vi "Write Move Enum_.vi"(8 "error in (no error)":errorcluster, 10 "Move Enum?":bool, 11 "Multi Column Listbox in":refnum<class "Multi Column Listbox.lvclass">) -> (0 "error out":errorcluster, 3 "Multi Column Listbox out":refnum<class "Multi Column Listbox.lvclass">)   [LabVIEW 2013]
uses:
  Multi Column Listbox.lvclass
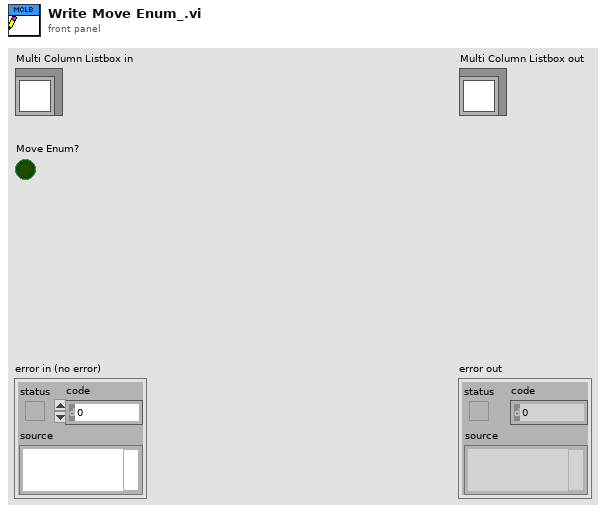
[diagram p1: front panel]
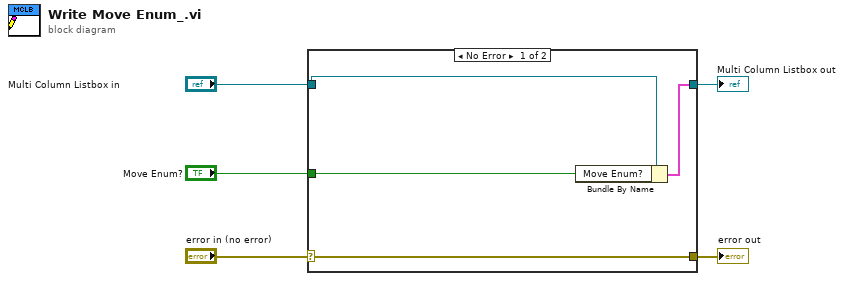
[diagram p0: block diagram]
diagram:
  n1 = case shown="No Error" "error in (no error)" {
    selector: "error in (no error)" -> [w9 w10]
    tunnel: [w9 w10] -> w4
    tunnel: [w7 w11] -> w2
    tunnel: "Multi Column Listbox in" -> [w8 w11]
    tunnel: "Move Enum?" -> [w6 _]
    frame No Error {
      n2 = Bundle By Name(cluster=w8, "Move Enum?"=w6) -> (w7:cluster{})
    }
    frame Error {
    }
  }
  "error out" <- w4
  "Multi Column Listbox out" <- w2
